vi "00 - Simple Debugging.vi"   [LabVIEW 2026]
uses:
  <vilib>/Utility/file.llb/Write Delimited Spreadsheet (DBL).vi
  <vilib>/Utility/sysdir.llb/System Directory Type.ctl
panel:
  # "Open Block Diagram to Debug Code\nCtl + E (instructions on diagram)"
types:
  T1 = typedef "System Directory Type.ctl" = i32
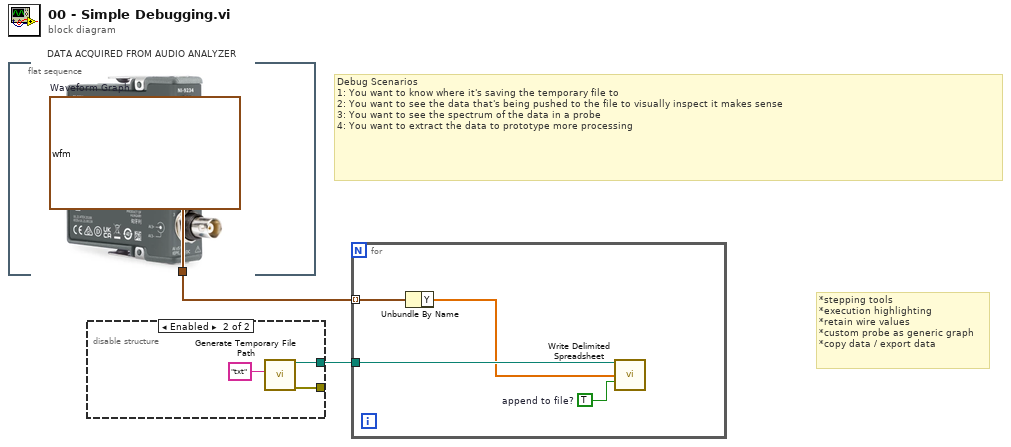
[diagram p0: block diagram]
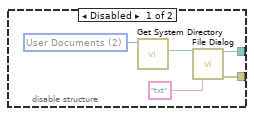
[diagram p2: hidden frame]
diagram:
  # "*stepping tools\n*execution highlighting\n*retain wire values\n*custom probe as generic graph\n*copy data / export data"
  # "Debug Scenarios\n1: You want to know where it's saving the temporary file to\n2: You want to see the data that's being pushed to the file to visually inspect it makes sense\n3: You want to see the spectrum of the data in a probe\n4: You want to extract the data to prototype more processing"
  n1 = flat-sequence "DATA ACQUIRED FROM AUDIO ANALYZER" {
    tunnel: [w3] -> w2
    frame #0 {
      w3 = waveform(dbl)[] [{"t0"=timestamp(0 s since 1904-01-01), "dt"=0.0002, "Y"=array[5000 elements]}, {"t0"=timestamp(0 s since 1904-01-01), "dt"=0.0002, "Y"=array[5000 elements]}]  # Waveform Graph
    }
  }
  n2 = disable-structure shown="Enabled" {
    disable-tunnel: [w8 w11] -> _
    disable-tunnel: [w5 w9] -> w1
    frame Disabled {
      w6 = T1 2 items=["User Home"=0, "User Desktop"=1, "User Documents"=2, "User Application Data"=3, "User Preferences"=4, "User Temporary"=5, "Public Documents"=6, "Public Application Data"=7, "Public Preferences"=8, "Public Cache"=13, "System Core Libraries"=9, "System Installed Libraries"=10, "Application Files"=11, "Boot Volume Root"=12] ("system directory type")
      n3 = call <vilib>:"Get System Directory.vi"("system directory type"=w6) -> ("system directory"=w7:path)  [unwired: 10 in]
      n4 = call "File Dialog"("start path"=w7, "pattern (all files)"="txt") -> ("selected path"=w5:path, "error out"=w8:errorcluster)  [unwired: 10 in, 2 out]
    }
    frame Enabled {
      n5 = call <vilib>:"Generate Temporary File Path.vi"("Temporary File Extension (tmp)"="txt" ("pattern (all files)")) -> ("error out"=w11:errorcluster, "Unique Temporary File Path"=w9:path)  [unwired: 9 in]
    }
  }
  n6 = for {
    tunnel: w2 -> [w13] mode=indexing
    tunnel: w1 -> [w15]
    w14 = TRUE  # append to file?
    n7 = Unbundle By Name(w13) -> ("Y"=w12:dbl[])
    n8 = call-poly <vilib>:"Write Delimited Spreadsheet.vi"("file path (dialog if empty)"=w15, "1D data"=w12, "append to file? (new file:F)"=w14) -> ()  [unwired: 11 in, 2 out]
  }
